vi "UpdateINIFile.vi"(5 "Files Generated by Build":path[](array[path]), 6 "Top Level/Always Included VIs":path[](array[path]), 7 "Destination Path":path, 8 "error in (no error)":errorcluster, 9 "Target Name":string, 10 "Build Specification Name":string, 11 "Project Path":path) -> (0 "error out":errorcluster)   [LabVIEW 2012]
uses:
  <vilib>/Utility/config.llb/Write Key (I32).vi
  <vilib>/Utility/config.llb/Write Key (Boolean).vi
  <vilib>/Utility/config.llb/NI_LVConfig.lvlib
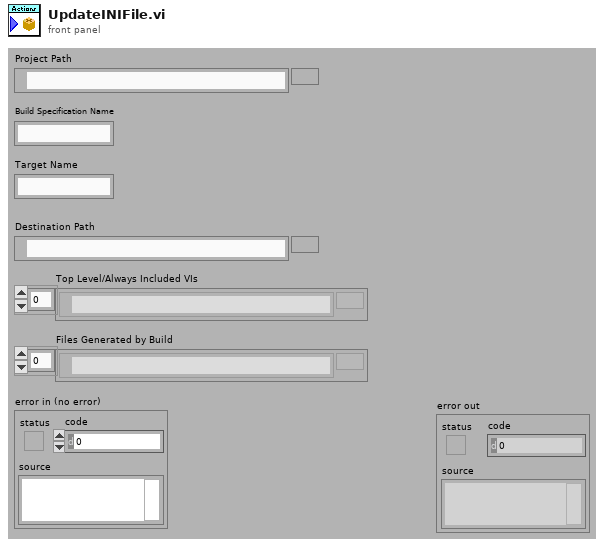
[diagram p1: front panel]
types:
  T1 = typedef "NI_LVConfig.lvlib/Config Data RefNum.ctl" = refnum<k1>
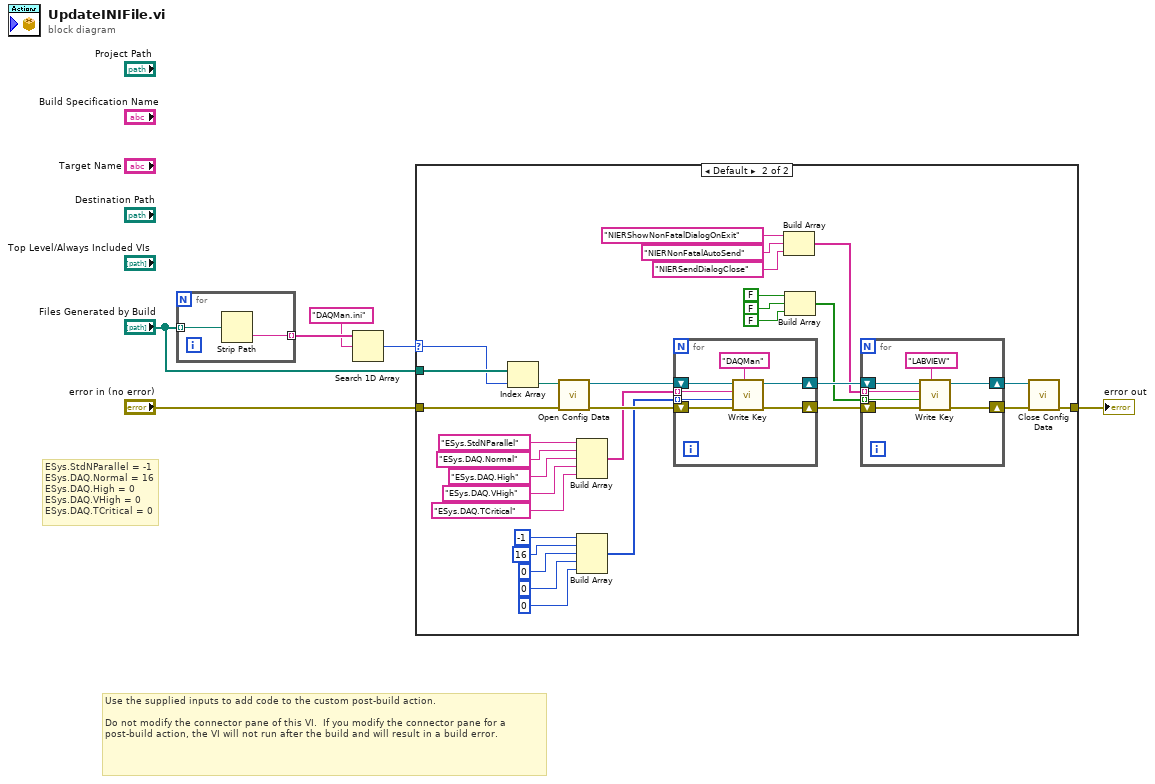
[diagram p0: block diagram]
diagram:
  # "ESys.StdNParallel = -1\nESys.DAQ.Normal = 16\nESys.DAQ.High = 0\nESys.DAQ.VHigh = 0\nESys.DAQ.TCritical = 0"
  # "Use the supplied inputs to add code to the custom post-build action.\n\nDo not modify the connector pane of this VI.  If you modify the connector pane for a post-build action, the VI will not run after the build and will result in a build error."
  n1 = for {
    tunnel: "Files Generated by Build" -> [w8] mode=indexing
    tunnel: [w7] -> w4 mode=indexing
    n2 = Strip Path(path=w8) -> (name=w7:string)  [unwired: 1 out]
  }
  n3 = Search 1D Array(1D array=w4, element="DAQMan.ini") -> (index of element=w1:i32)  [unwired: 1 in]
  n4 = case shown="Default" w1 {
    selector: w1 -> [_ w22]
    tunnel: "error in (no error)" -> [w9 w40]
    tunnel: [w9 w38] -> w5
    tunnel: "Files Generated by Build" -> [_ w24]
    frame -1 {
    }
    frame Default {
      n5 = Index Array(array=w24, index=w22) -> (element=w23:path)
      n6 = call <vilib>:"Open Config Data.vi"("error in (no error)"=w40, "configuration file path"=w23) -> ("error out"=w39:errorcluster, "refnum"=w27:T1)  [unwired: 7 in, 1 out]
      n7 = Build Array("ESys.StdNParallel", "ESys.DAQ.Normal", "ESys.DAQ.High", "ESys.DAQ.VHigh", "ESys.DAQ.TCritical") -> (w26:string[])
      n8 = Build Array(-1, 16, 0, 0, 0) -> (w25:i32[])
      n9 = for {
        shift-right: [w53] -> w20
        shift-left: w39 -> [w54]
        shift-right: [w51] -> w21
        shift-left: w27 -> [w52]
        tunnel: w26 -> [w49] mode=indexing
        tunnel: w25 -> [w48] mode=indexing
        n10 = call-poly <vilib>:"Write Key.vi"("section"="DAQMan", "error in (no error)"=w54, "value"=w48, "key"=w49, "refnum"=w52) -> ("error out"=w53:errorcluster, "refnum out"=w51:T1)  [unwired: 4 in, 1 out]
      }
      n11 = Build Array("NIERShowNonFatalDialogOnExit", "NIERNonFatalAutoSend", "NIERSendDialogClose") -> (w14:string[])
      n12 = Build Array(FALSE, FALSE, FALSE) -> (w10:bool[])
      n13 = for {
        shift-right: [w46] -> w18
        shift-left: w20 -> [w47]
        shift-right: [w44] -> w19
        shift-left: w21 -> [w45]
        tunnel: w14 -> [w42] mode=indexing
        tunnel: w10 -> [w41] mode=indexing
        n14 = call-poly <vilib>:"Write Key.vi"("section"="LABVIEW", "error in (no error)"=w47, "value"=w41, "key"=w42, "refnum"=w45) -> ("error out"=w46:errorcluster, "refnum out"=w44:T1)  [unwired: 4 in, 1 out]
      }
      n15 = call <vilib>:"Close Config Data.vi"("error in (no error)"=w18, "refnum"=w19) -> ("error out"=w38:errorcluster)  [unwired: 8 in, 1 out]
    }
  }
  "error out" <- w5
